vi "Comprehensive Sanity Check.vi"(8 "error in (no error)":errorcluster) -> (0 "error out":errorcluster, 2 "Passed?":bool)   [LabVIEW 2013]
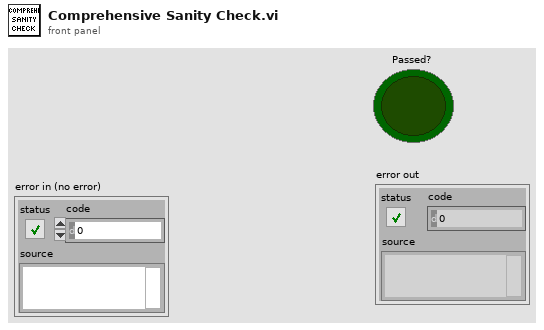
[diagram p1: front panel]
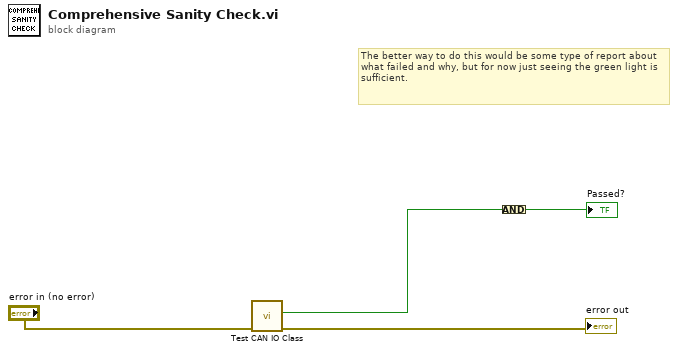
[diagram p0: block diagram]
diagram:
  # "The better way to do this would be some type of report about what failed and why, but for now just seeing the green light is sufficient."
  n1 = call "Test CAN IO Class.vi"("error in (no error)"="error in (no error)") -> ("error out"=→"error out":errorcluster, "Passed?"=w1:bool)  [unwired: 9 in]
  n2 = Compound Arithmetic op=AND(w1) -> (→"Passed?":bool)
